vi "Get Measurement Paths.vi"(0 "measurement path":path, 5 "measurement plug-ins":string[][](array[string]), 7 "measurement folder selected?":bool, 11 "error in":errorcluster) -> (4 "measurement path array":path[](array[path]), 15 "error out":errorcluster)   [LabVIEW 2021, in "Path Functions.lvlib"]
uses:
  Path Functions.lvlib
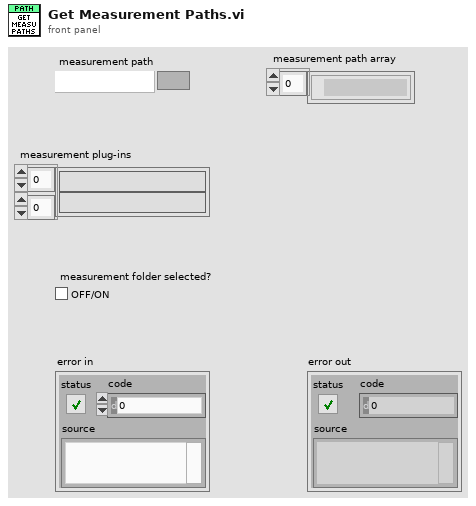
[diagram p1: front panel]
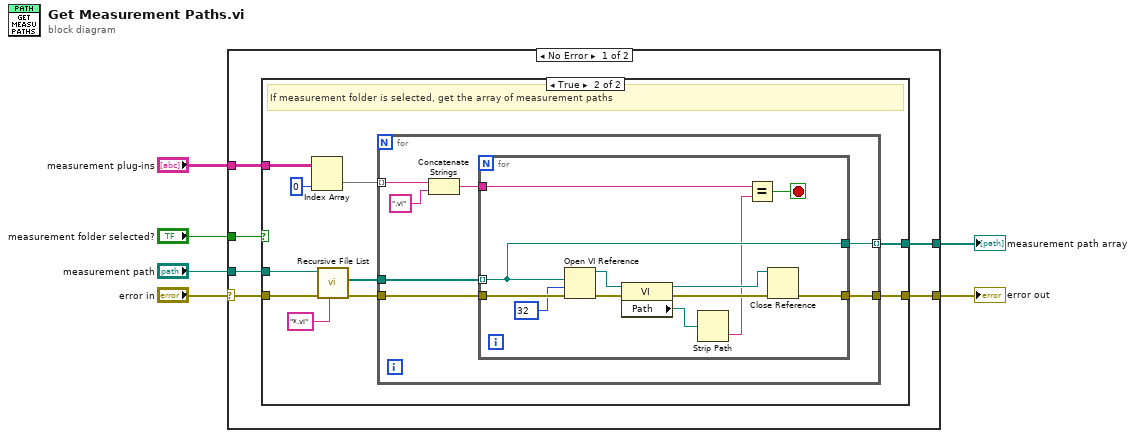
[diagram p0: block diagram]
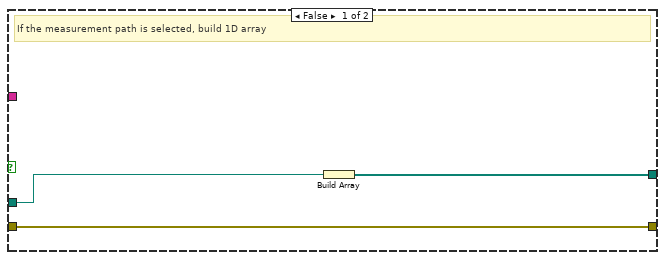
[diagram p2: hidden frame]
diagram:
  n1 = case shown="No Error" "error in" {
    selector: "error in" -> [w10 w45]
    tunnel: [w11 w45] -> w1
    tunnel: "measurement plug-ins" -> [w12 _]
    tunnel: "measurement path" -> [w7 _]
    tunnel: [w9 _] -> w2
    tunnel: "measurement folder selected?" -> [w8 _]
    frame No Error {
      n2 = case shown="True" w8 {
        tunnel: w7 -> [w13 w24]
        tunnel: w12 -> [_ w23]
        tunnel: [w15 w18] -> w11
        tunnel: w10 -> [w15 w25]
        tunnel: [w14 w17] -> w9
        frame False {
          # "If the measurement path is selected, build 1D array"
          n3 = Build Array(w13) -> (w14:path[])
        }
        frame True {
          # "If measurement folder is selected, get the array of measurement paths"
          n4 = Index Array(array=w23, index (col)=0 ("disabled index (col)")) -> (element=w21:string[])  [unwired: 1 in]
          n5 = call <vilib>:"Recursive File List.vi"("pattern"="*.vi", "error in (no error)"=w25, "Folder Path"=w24) -> ("error out"=w19:errorcluster, "All Files in Dir"=w20:path[])  [unwired: 4 in, 3 out]
          n6 = for {
            tunnel: w21 -> [w32] mode=indexing
            tunnel: w20 -> [w30]
            tunnel: w19 -> [w29]
            tunnel: [w27] -> w18
            tunnel: [w28] -> w17 mode=indexing
            n7 = Concatenate Strings(w32, ".vi" ("string")) -> (w31:string)
            n8 = for {
              tunnel: w31 -> [w40]
              tunnel: w30 -> [w39] mode=indexing
              tunnel: w29 -> [w44]
              tunnel: [w37] -> w27
              tunnel: [w39] -> w28
              stop <- w35 stop-if-true
              n9 = Open VI Reference(vi path=w39, options=32, error in (no error)=w44) -> (vi reference=w41:refnum<vi>, error out=w42:errorcluster)  [unwired: 3 in]
              n10 = property class="VI"(reference=w41, error in=w42) -> (reference out=w36:refnum<vi>, error out=w38:errorcluster, "Path"=w34:path)
              n11 = Strip Path(path=w34) -> (name=w33:string)  [unwired: 1 out]
              n12 = Equal?(x=w40, y=w33) -> (x = y?=w35:bool)
              n13 = Close Reference(reference=w36, error in (no error)=w38) -> (error out=w37:errorcluster)
            }
          }
        }
      }
    }
    frame Error {
    }
  }
  "error out" <- w1
  "measurement path array" <- w2
